vi "set_cycles.vi"(8 "error in":errorcluster, 10 "Cycles":u16, 11 "FPGAWrapperRK110909Throughput in":refnum<class "FPGAWrapperRK110909Throughput.lvclass">) -> (0 "error out":errorcluster, 3 "FPGAWrapperRK110909Throughput in 2":refnum<class "FPGAWrapperRK110909Throughput.lvclass">)   [LabVIEW 2010, in "FPGAWrapperRK110909Throughput.lvclass"]
uses:
  FPGAWrapperRK110909Throughput.lvclass
  <vilib>/rvi/interface/nirviReadWriteControl/nirviReadWriteControl.xnode
  FPGA_reference.ctl
  <vilib>/rvi/interface/common/niFpgaNodeNameForErrorReporting.ctl
  <vilib>/rvi/errors/niLvFpgaWhatHappensToTopLevelVI.ctl
  <vilib>/Utility/error.llb/Error Cluster From Error Code.vi
  <vilib>/rvi/errors/niLvFpgaAdjustHostInterfaceError.vi
  NiFpgaLv.dll
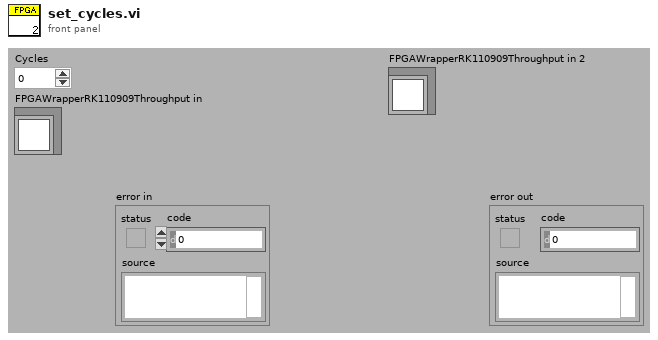
[diagram p1: front panel]
types:
  T1 = typedef "niFpgaNodeNameForErrorReporting.ctl" = enum16{"Open FPGA VI Reference", "Read/Write Control", "Invoke Method: Abort", "Invoke Method: Acknowledge IRQ", "Invoke Method: Download", "Invoke Method: FIFO.Configure", "Invoke Method: FIFO.Read", "Invoke Method: FIFO.Start", "Invoke Method: FIFO.Stop", "Invoke Method: FIFO.Write", "Invoke Method: Reset", "Invoke Method: Run", "Invoke Method: Wait on IRQ", "Close FPGA VI Reference"}
  T2 = typedef "niLvFpgaWhatHappensToTopLevelVI.ctl" = enum16{"top level VI scripted behind XNode", "top level VI inlined behind XNode"}
  T3 = typedef "FPGAWrapperRK110909Throughput.lvclass/FPGA_reference.ctl" = refnum<k20>
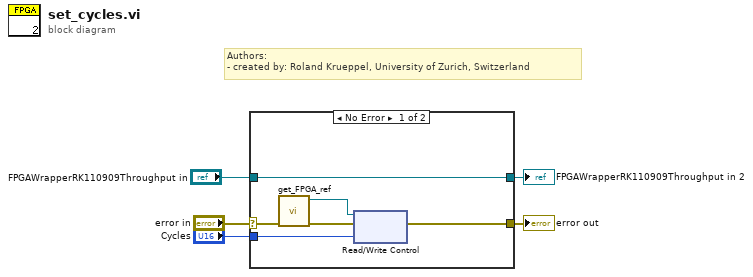
[diagram p0: block diagram]
diagram:
  # "Authors: \n- created by: Roland Krueppel, University of Zurich, Switzerland"
  n1 = case shown="No Error" "error in" {
    selector: "error in" -> [w11 w51]
    tunnel: [w9 w51] -> w4
    tunnel: "Cycles" -> [w7 _]
    tunnel: "FPGAWrapperRK110909Throughput in" -> [w6 w50]
    tunnel: [w6 w50] -> w1
    frame No Error {
      n2 = call "get_FPGA_ref.vi"("error in"=w11) -> ("error out"=w10:errorcluster, "FPGA Reference"=w8:T3)  [unwired: 8 in, 1 out]
      n3 = xnode "Read/Write Control"("FPGA VI Reference In"=w8, "error in"=w10, "Cycles"=w7) -> ("error out"=w9:errorcluster)  [unwired: 1 out]
    }
    frame Error {
    }
  }
  "error out" <- w4
  "FPGAWrapperRK110909Throughput in 2" <- w1
